vi "Message Type.vi"(4 "Group Type":T1) -> (7 "type":string)   [LabVIEW 2020, in "VolatusTelemetry.lvlib"]
uses:
  VolatusTelemetry.lvlib
  VolatusConfig/Group Type.ctl
  VolatusConfig/VolatusConfig.lvlib
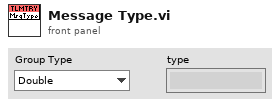
[diagram p1: front panel]
types:
  T1 = typedef "VolatusConfig.lvlib/Group Type.ctl" = enum16{"Double", "Bool", "String"}
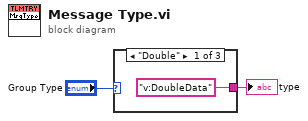
[diagram p0: block diagram]
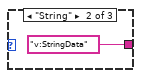
[diagram p2: hidden frame]
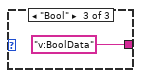
[diagram p3: hidden frame]
diagram:
  n1 = case shown="\"Double\"" "Group Type" {
    tunnel: ["v:DoubleData" ("type") "v:StringData" ("type") "v:BoolData" ("type")] -> w1
    frame "Double" {
    }
    frame "String" {
    }
    frame "Bool" {
    }
  }
  "type" <- w1
